vi "Get Table Columns Name.vi"(8 "error in (no error)":errorcluster, 10 "TableName":string, 11 "HostDB in":refnum<class "SQLite.lvclass">) -> (0 "error out":errorcluster, 1 "DB Data Type":T1(array[ring]), 2 "Table_ColunmsList":string[](array[string]), 3 "HostDB out":refnum<class "SQLite.lvclass">, 4 "TableName List":string[](array[string]))   [LabVIEW 2017, in "SQLite.lvclass"]
uses:
  SQLite.lvclass
  \\vmware-host\Shared Folders/D/Dev/NJAL/OP140/OP140_NJAL_valve_EOL_Test_20210806/Source_Public/DataBase/Top DB/TopDBClass.lvclass
  <userlib>/LabSQL/LabSQL.lvlib
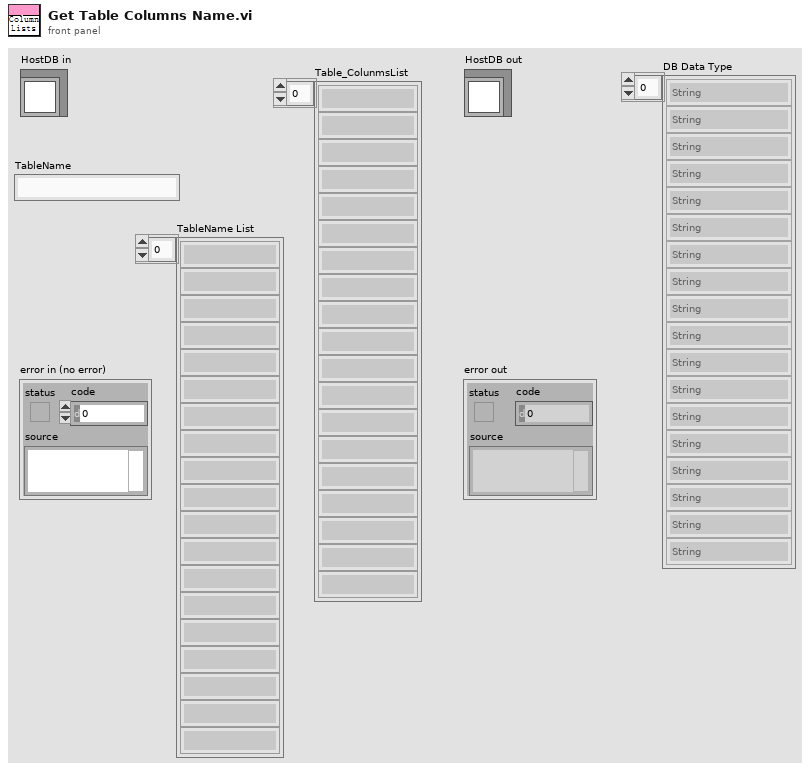
[diagram p1: front panel]
types:
  T1 = enum16{"String", "Long (I32)", "Single (SGL)", "Double (DBL)", "Date/Time", "Binary"}[]
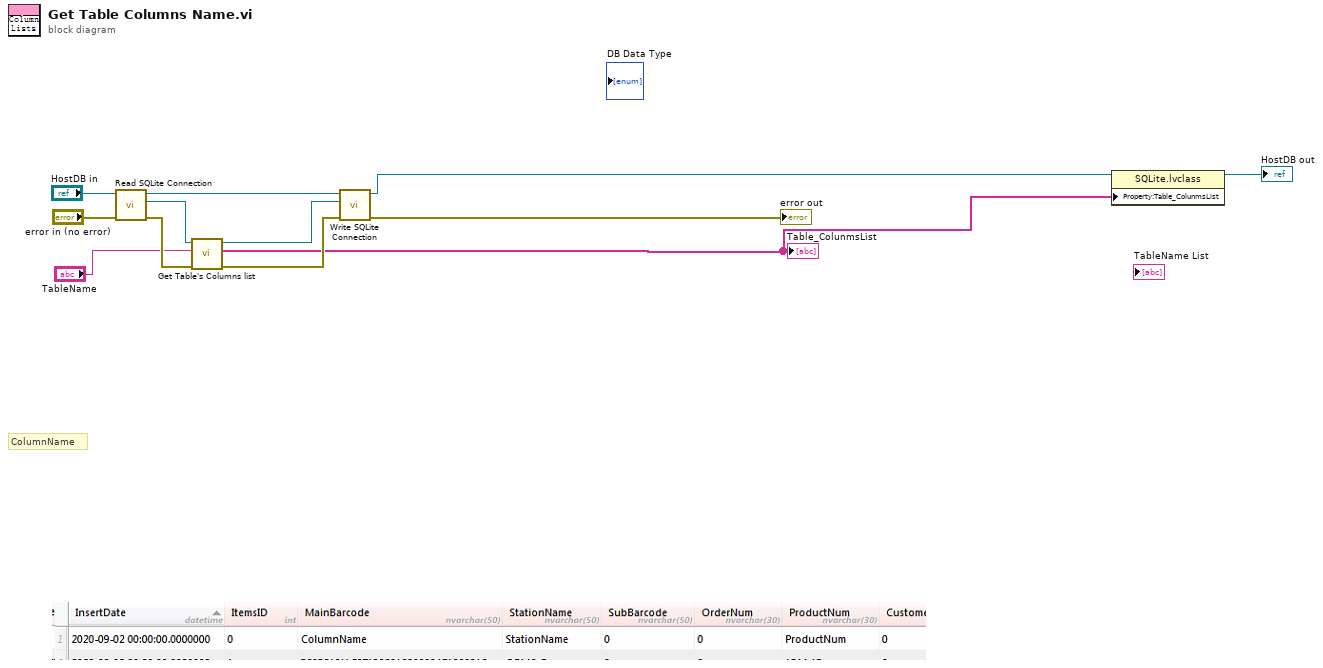
[diagram p0: block diagram]
diagram:
  # "ColumnName"
  n1 = call-dynamic "Read SQLite Connection.vi"("error in (no error)"="error in (no error)", "SQLite in"="HostDB in") -> ("error out"=w10:errorcluster, "SQLite.lvlib:Connection"=w11:refnum<class "Connection.lvclass">, "SQLite out"=w8:refnum<class "SQLite.lvclass">)  [unwired: 7 in]
  n2 = call <userlib>:"Get Table's Columns list.vi"("error in (no error)"=w10, "TabelName"="TableName", "SQLite Connection in"=w11) -> ("error out"=w9:errorcluster, "Column Names"=w1:string[], "SQLite Connection out"=w5:refnum<class "Connection.lvclass">)  [unwired: 5 in, 1 out]
  "Table_ColunmsList" <- w1
  n3 = call-dynamic "Write SQLite Connection.vi"("error in (no error)"=w9, "SQLite.lvlib:Connection"=w5, "SQLite in"=w8) -> ("error out"=→"error out":errorcluster, "SQLite out"=w4:refnum<class "SQLite.lvclass">)  [unwired: 7 in]
  n4 = property class="SQLite.lvclass"(reference=w4, "Property:Table_ColunmsList"=w1) -> (reference out=→"HostDB out":refnum<class "SQLite.lvclass">)  [unwired: 1 in, 1 out]
